vi "Read VI Refnum Lifetime.vi"(8 "error in (no error)":errorcluster, 11 "Async Message in":refnum<class "Async Message.lvclass">) -> (0 "error out":errorcluster, 2 "VI Refnum Lifetime":T1, 3 "Async Message out":refnum<class "Async Message.lvclass">)   [LabVIEW 2023, in "Async Methods Actor.lvlib" / "Async Message.lvclass"]
doc: "This enumeration can take values \"Destroy on Exit\", \" Destroy on Actor Exit \", and “Destroy on Application Exit”. This enumeration dictates the lifetime strategy adopted for the VI Refnum of the Async Method. In the first case the \"Async Methods Actor\" destroys the reference as soon as the Async Method Exits, in the second case the VI Refnums will be destroyed once the “Async Method Actor” exits, while in the last case, VI Refnums are never destroyed. “Destroy on Exit” is the default option when unwired. The motivation for this setting is related to the required lifetimes of the Refnums (e.g. notifier’s references) created within the Async Method. This lifetime is the same as the VI Refnum lifetime, hence if we want they outlive the execution of the Async Method we have to set it to either “Destroy on Actor Exit” or “Destroy on Application Exit”. This option applies only to Async Methods called with the “Call and Collect” option."
uses:
  Async Message.lvclass
  Async Methods Actor/VI Refnum Lifetime.ctl
  Async Message.lvclass/Async Message.ctl
  Async Methods Actor/Async Methods Actor.lvclass
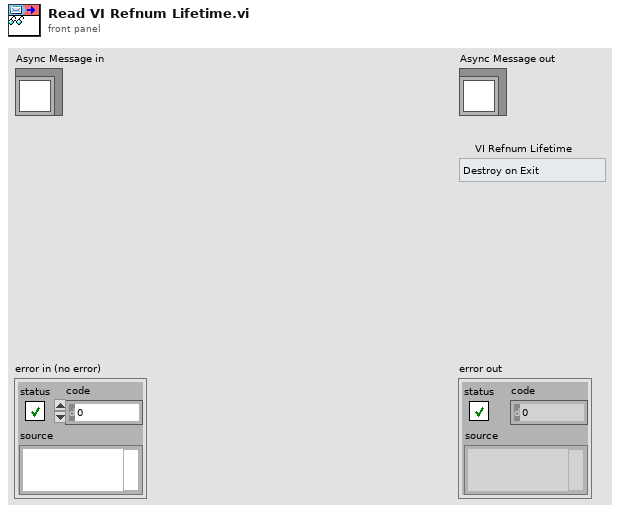
[diagram p1: front panel]
types:
  T1 = typedef "Async Methods Actor.lvlib/Async Methods Actor.lvclass/VI Refnum Lifetime.ctl" = enum16{"Destroy on Exit", "Destroy on Actor Exit", "Destroy on Application Exit"}
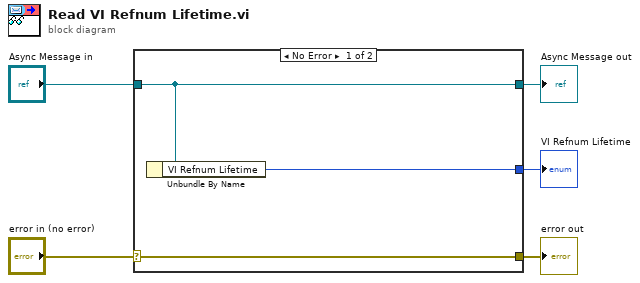
[diagram p0: block diagram]
diagram:
  n1 = case shown="No Error" "error in (no error)" {
    selector: "error in (no error)" -> [w8 w9]
    tunnel: [w8 w9] -> w4
    tunnel: [w7 w10] -> w2
    tunnel: "Async Message in" -> [w7 w10]
    tunnel: [w6 _] -> w1
    frame No Error {
      n2 = Unbundle By Name(w7) -> ("VI Refnum Lifetime"=w6:T1)
    }
    frame Error {
    }
  }
  "error out" <- w4
  "Async Message out" <- w2
  "VI Refnum Lifetime" <- w1
